vi "Configure UI.vi"(8 "error in (no error)":errorcluster, 10 "Project In":refnum<class "Project.lvclass">, 11 "SerializableObject in":refnum<class>) -> (0 "error out":errorcluster, 3 "SerializableObject out":refnum<class>)   [LabVIEW 2015, in "SerializableObject.lvclass"]
uses:
  SerializableObject.lvclass
  Project.lvclass
  CONFIGURE_UI_STATE.ctl
  Editor/Editor.lvclass
panel:
  in  "Boolean":bool
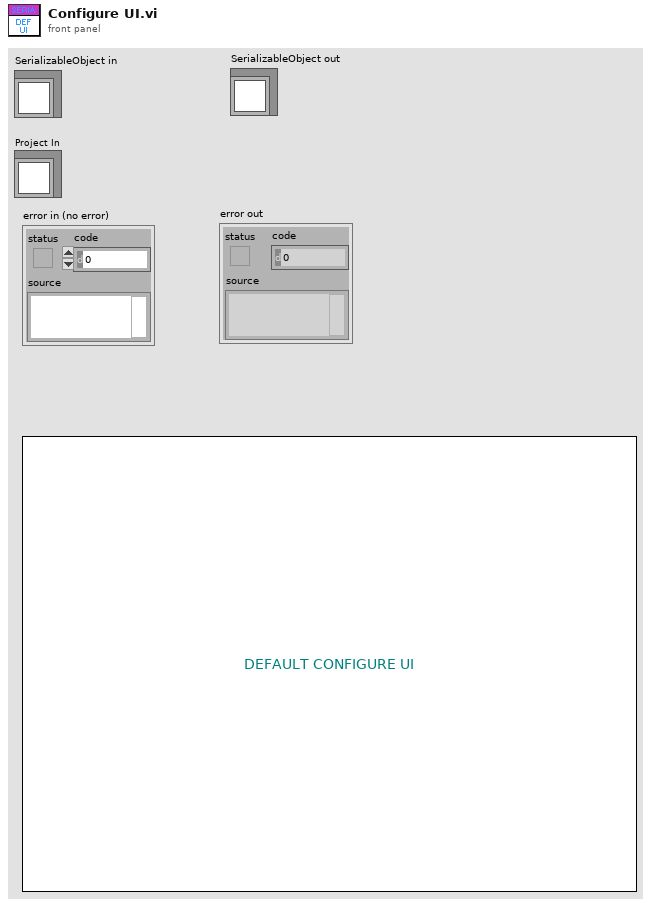
[diagram p1: front panel]
types:
  T1 = typedef "Editor.lvclass/CONFIGURE_UI_STATE.ctl" = enum16{"UI_LOOP", "INIT", "END", "CHANGE_PANEL"}
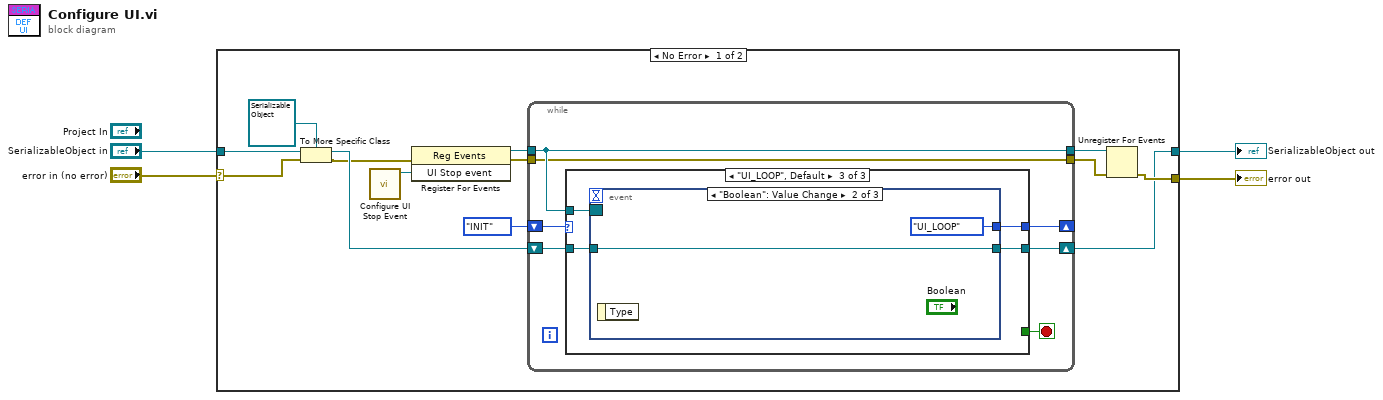
[diagram p0: block diagram]
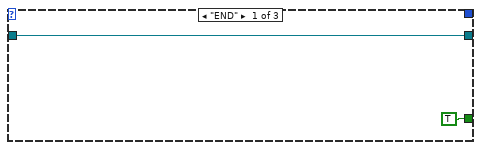
[diagram p2: hidden frame]
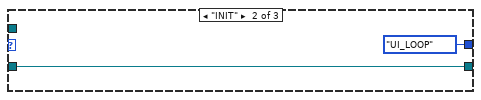
[diagram p3: hidden frame]
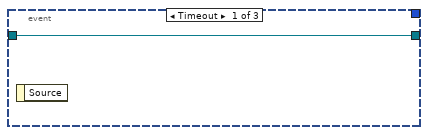
[diagram p4: hidden frame]
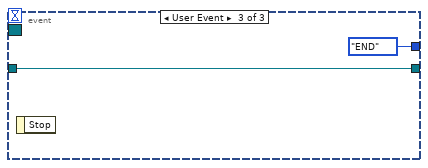
[diagram p5: hidden frame]
diagram:
  n1 = case shown="No Error" "error in (no error)" {
    selector: "error in (no error)" -> [w15 w39]
    tunnel: [w9 w39] -> w3
    tunnel: "SerializableObject in" -> [w17 w38]
    tunnel: [w8 w38] -> w1
    frame No Error {
      n2 = To More Specific Class(target class=refnum<class "SerializableObject.lvclass"> refnum ("ConfigureableObject in"), reference=w17, error in=w15) -> (specific class reference=w7:refnum<class "SerializableObject.lvclass">, error out=w5:errorcluster)
      n3 = call "Configure UI Stop Event.vi"() -> ("UI Stop event"=w6:refnum<user-event>)  [unwired: 11 in]
      n4 = register-events(error in=w5, w6) -> (reference out=w10:refnum<event-registration>, error out=w12:errorcluster)  [unwired: 1 in]
      n5 = while {
        tunnel: w10 -> [w24]
        tunnel: [w24] -> w11
        tunnel: w12 -> [w23]
        tunnel: [w23] -> w13
        shift-right: [w21] -> w8
        shift-left: w7 -> [w22]
        shift-right: [w19] -> _
        shift-left: CONFIGURE_UI_STATE."INIT" -> [w20]
        stop <- w18 stop-if-true
        n6 = case shown="\"UI_LOOP\", Default" w20 {
          tunnel: w24 -> [_ _ w32]
          tunnel: w22 -> [w25 w27 w31]
          tunnel: [w25 w27 w30] -> w21
          tunnel: [_ CONFIGURE_UI_STATE."UI_LOOP" w29] -> w19
          tunnel: [TRUE _ _] -> w18
          frame "END" {
          }
          frame "INIT" {
          }
          frame "UI_LOOP", Default {
            n7 = event shown="[1] \"Boolean\": Value Change" {
              selector: w32 -> [_ _ _]
              dyn-events: _ -> [_ _ _]
              timeout: _ -> [_ _ _]
              tunnel: w31 -> [w33 w35 w37]
              tunnel: [w33 w35 w37] -> w30
              tunnel: [_ CONFIGURE_UI_STATE."UI_LOOP" CONFIGURE_UI_STATE."END"] -> w29
              event Timeout {
                n8 = event-data() -> ()  [unwired: 1 in, 1 out]
              }
              event "Boolean": Value Change {
                n9 = event-data() -> ()  [unwired: 1 in, 1 out]
              }
              event User Event {
                n10 = event-data() -> ()  [unwired: 1 in, 1 out]
              }
            }
          }
        }
      }
      n11 = Unregister For Events(event registration refnum=w11, error in=w13) -> (error out=w9:errorcluster)
    }
    frame Error {
    }
  }
  "error out" <- w3
  "SerializableObject out" <- w1
